vi "LDA_cold_wire_Corr_with_ Displacement.vi"() -> (5 "Plug in titles":string[](array[string]), 7 "Plug in values":string[](array[string]))   [LabVIEW 2016]
uses:
  Globals/Meas_global.vi
  Globals/LDA_meas_global_1.vi
panel:
  in  "Cold Wire":i32=2
  in  "X Displacement (mm)":dbl=4.0
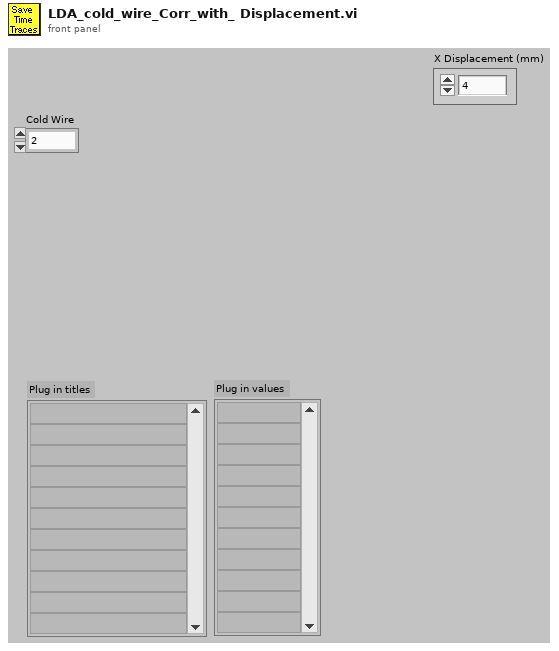
[diagram p1: front panel]
types:
  T1 = typedef "Analysis_info_cluster.ctl" = cluster{"Colour":u32, "Inst type":T2, "Inst name":string, "Symbol":string, "Code name":string, "Extra Info":string, "Inst Array":T3, "Extra Titles":string[], "Extra Values":string[], "U":dbl, "u^2":dbl, "u^3":dbl, "u^4":dbl, "Skew_u":dbl, "Kurt_u":dbl, "Sd Error in Mean":dbl, "% u'/U":dbl, "X":dbl, "Y":dbl, "Z":dbl, "Timescale integral Estimate":dbl, "Sd Error in Variance":dbl, "Calib File":path, "Calib Constants":dbl[], "Output Position":bool, "Full Stats":bool, "Av Sampling Rate":dbl, "Av No of Samples":dbl, "Total Meas Time (s)":dbl, "ADAM Ch Name":string, "Max value":dbl, "Min value":dbl}
  T2 = typedef "Inst_type.ctl" = enum16{"Propeller anemometer", "Raw voltage", "Pressure Transducer", "Pitot-static tube", "Preston tube", "Hot wire", "Cross wire 1", "Cross wire 2", "Generic Linear", "Generic Polynomial", "Generic BackPoly", "Fast FID", "Thermocouple", "Cold wire", "Pulsed Wire", "LDA Vel", "LDA Tran time", "LDA Arr time", "Microphone"}
  T3 = typedef "Instrument_Array.ctl" = enum16{"PWA", "LDA", "Analogue"}
  T4 = typedef "Time_Trace_Cluster.ctl" = cluster{"Weighting":dbl[], "Time (s)":dbl[], "Voltage":dbl[], "Eng Values":dbl[]}
  T5 = typedef "Shift_Cluster.ctl" = cluster{"Stats":dbl[], "Spectra_Auto":dbl[], "Histogram":dbl[], "Hist Max":dbl, "Hist Min":dbl, "No of Samples":i32, "No in plume":i32, "Weight sum":dbl, "No Of Hist bins":i32, "TimeTrace Max":dbl, "Time Trace Min":dbl, "Trace St Deviation":dbl}
  T6 = typedef "Correlation_cluster1.ctl" = cluster{"U inst":string, "uw":dbl, "u^2w":dbl, "uw^2":dbl, "uw/u'w'":dbl, "W inst":string, "uw^3":dbl, "u^3w":dbl, "u^2w^2":dbl, "Index U":i32, "Index W":i32, "Error info":string[]}
  T7 = typedef "Cross_Moments_Shift_Cluster.ctl" = cluster{"Stats":dbl[], "Resampled No of Samples":i32, "Resampled delta T":dbl, "Cross Correlation":dbl[]}
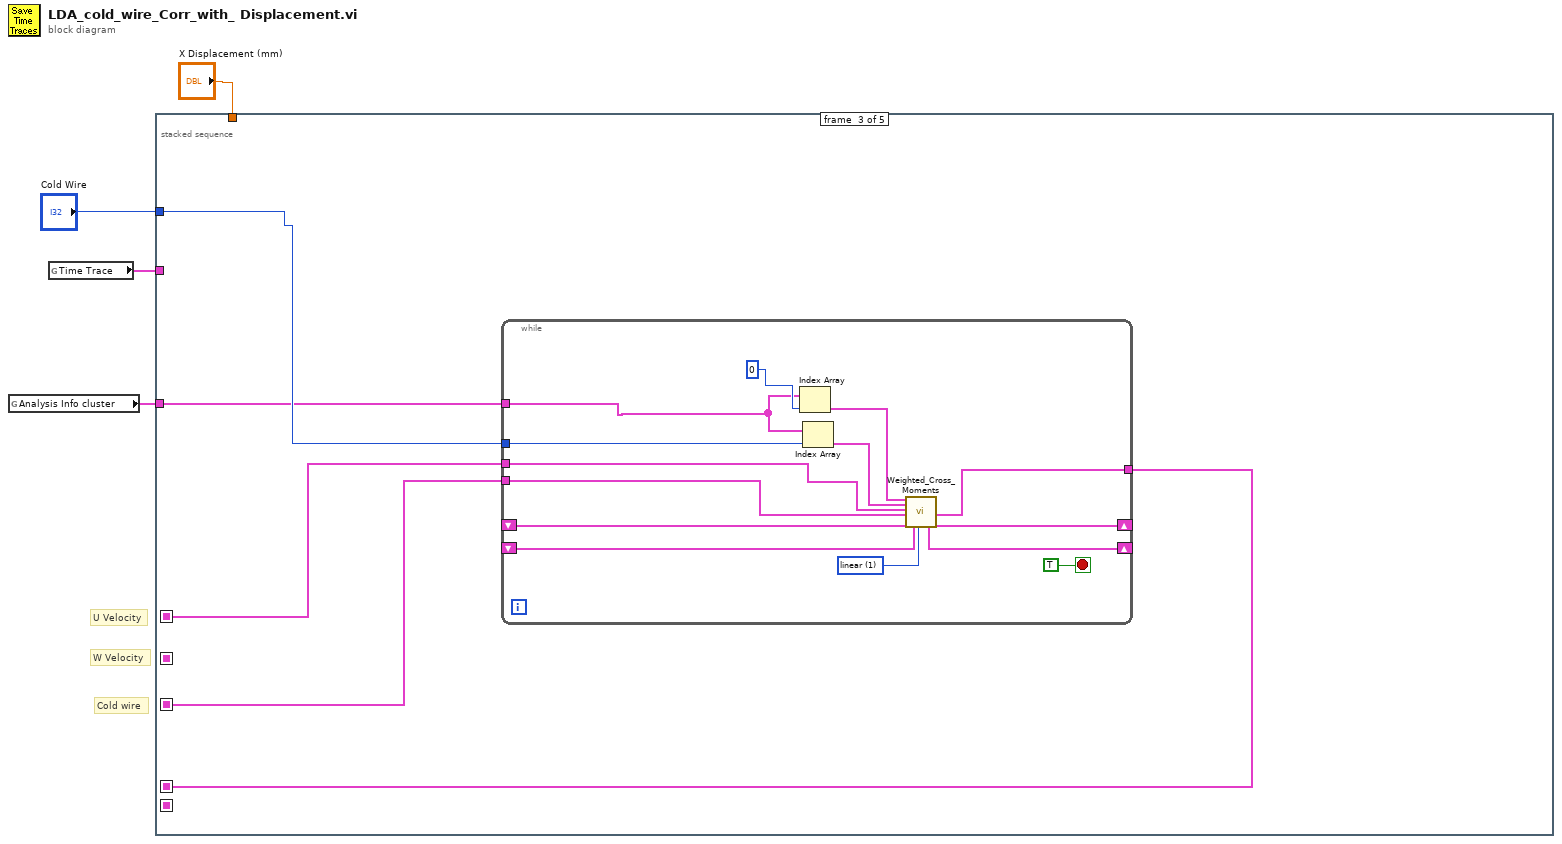
[diagram p0: block diagram]
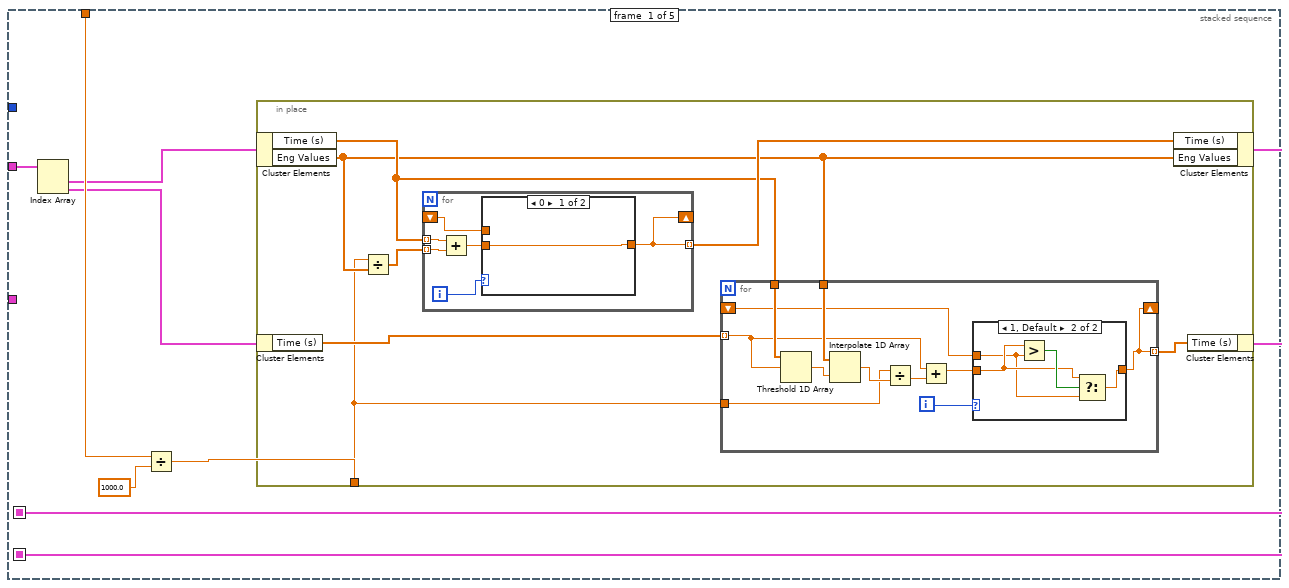
[diagram p2: hidden frame]
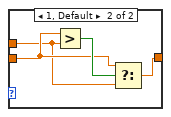
[diagram p3: hidden frame]
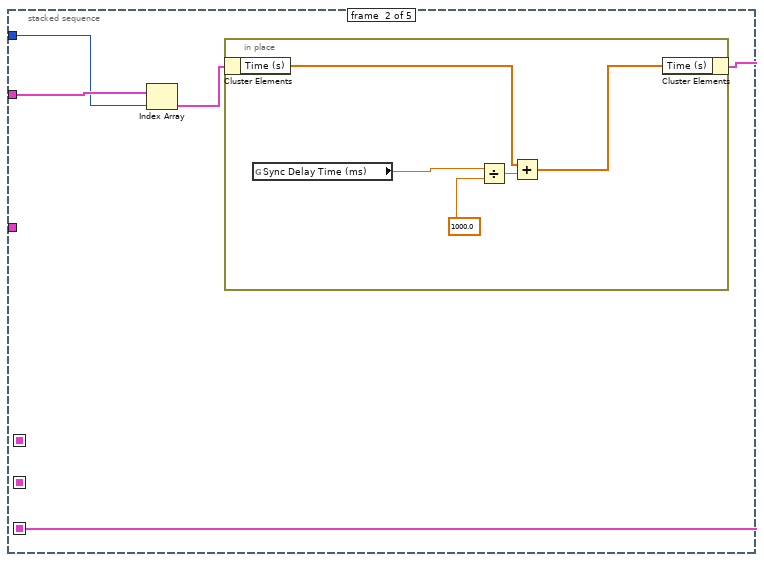
[diagram p5: hidden frame]
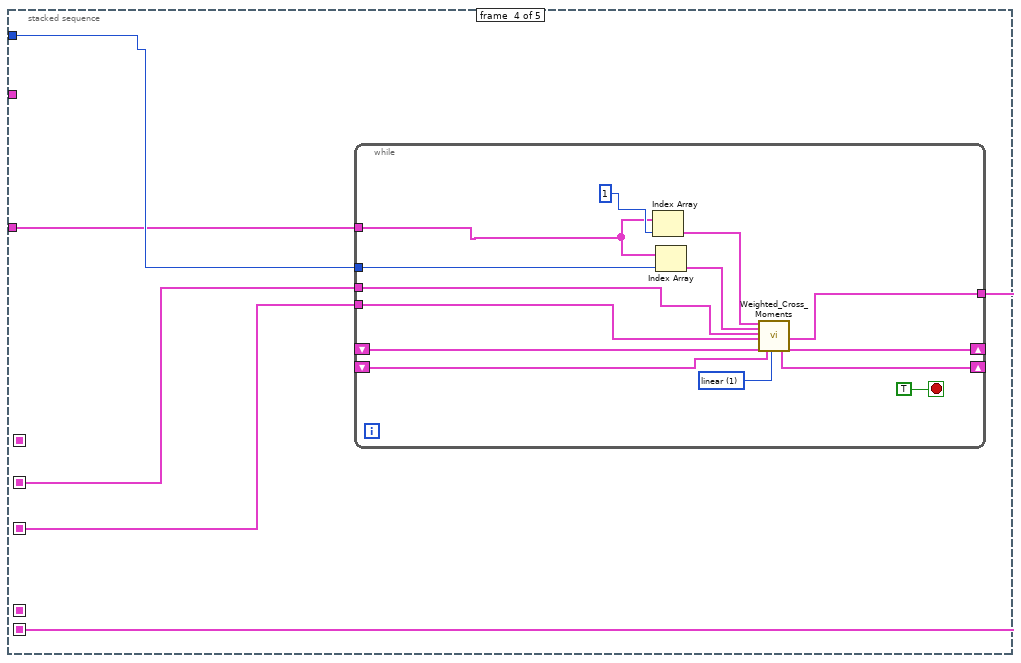
[diagram p6: hidden frame]
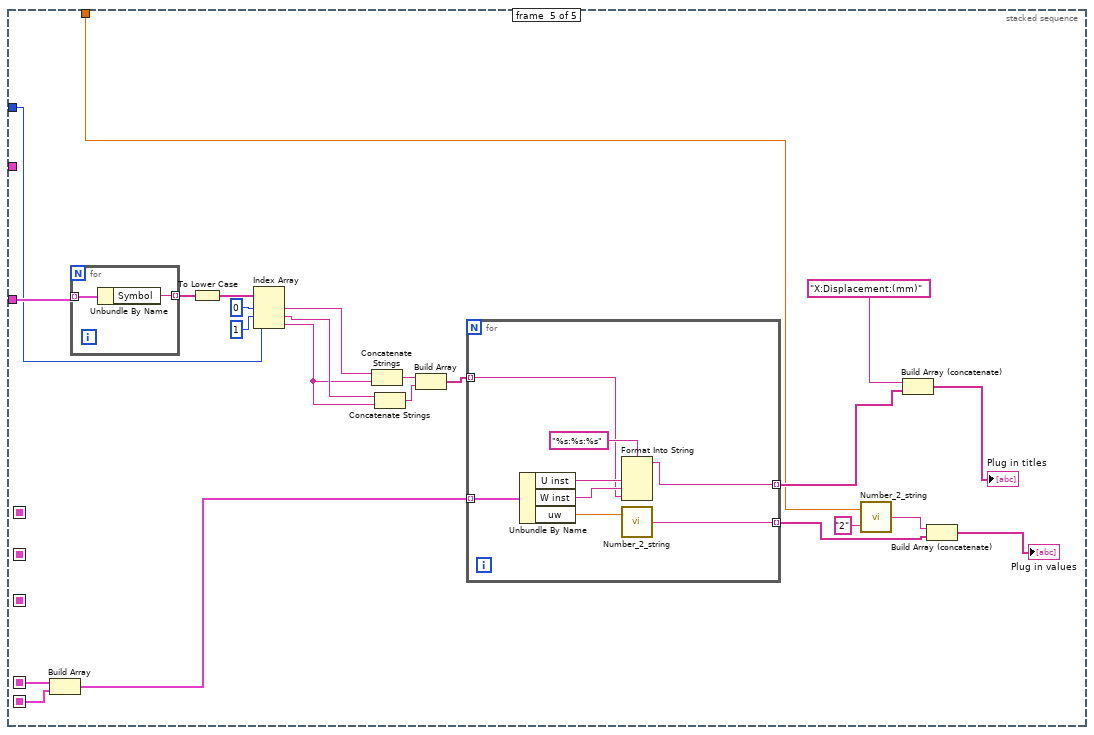
[diagram p7: hidden frame]
diagram:
  # "W Velocity"
  # "Cold wire"
  # "U Velocity"
  n1 = global read "Meas_global.vi" "Analysis Info cluster"() -> (w1:T1[])
  n2 = global read "Meas_global.vi" "Time Trace"() -> (w3:T4[])
  n3 = stacked-sequence {
    seq-local: [w7 _ _ _ _] -> [_ _ w60 _ _]
    seq-local: [_ w48 _ _ _] -> [_ _ w59 w79 _]
    seq-local: [_ _ w57 _ _] -> [_ _ _ _ w115]
    seq-local: [w5 _ _ _ _] -> [_ _ _ w76 _]
    seq-local: [_ _ _ w75 _] -> [_ _ _ _ w116]
    tunnel: "X Displacement (mm)" -> [w12 _ _ _ w95]
    tunnel: w3 -> [w10 w50 _ _ _]
    tunnel: "Cold Wire" -> [_ w47 w58 w78 w110]
    tunnel: w1 -> [_ _ w56 w77 w113]
    frame #0 {
      n4 = Index Array(array=w10) -> (element #1=w9:T4, element #2=w6:T4)  [unwired: 2 in]
      n5 = Divide(x=w12, y=1000.0) -> (x/y=w8:dbl)
      n6 = in-place {
        in-place-border: w8 -> [w15]
        n7 = in-place-cluster #1(w9) -> ("Time (s)"=w18:dbl[], "Eng Values"=w16:dbl[])
        n8 = in-place-cluster #2(w6) -> ("Time (s)"=w17:dbl[])
        n9 = Divide(x=w15, y=w16) -> (x/y=w13:dbl[])
        n10 = for {
          tunnel: w13 -> [w25] mode=indexing
          tunnel: [w21] -> w19 mode=indexing
          tunnel: w18 -> [w24] mode=indexing
          shift-right: [w21] -> _
          shift-left: _ -> [w22]
          i -> [w20]
          n11 = Add(x=w24, y=w25) -> (x+y=w23:dbl)
          n12 = case shown="0" w20 {
            tunnel: w23 -> [w26 w29]
            tunnel: w22 -> [_ w28]
            tunnel: [w26 w27] -> w21
            frame 0 {
            }
            frame 1, Default {
              n13 = Greater?(x=w29, y=w28) -> (0:w30:bool)
              n14 = Select(t=w29, s=w30, f=w28) -> (s? t:f=w27:dbl)
            }
          }
        }
        n15 = for {
          tunnel: w18 -> [w41]
          tunnel: w17 -> [w35] mode=indexing
          tunnel: w16 -> [w40]
          tunnel: w15 -> [w37]
          tunnel: [w32] -> w14 mode=indexing
          shift-right: [w32] -> _
          shift-left: _ -> [w33]
          i -> [w31]
          n16 = Threshold 1D Array(2:w35, 3:w41) -> (0:w39:dbl)  [unwired: 1 in]
          n17 = Interpolate 1D Array(1:w39, 2:w40) -> (0:w38:dbl)
          n18 = Divide(x=w37, y=w38) -> (x/y=w36:dbl)
          n19 = Add(x=w35, y=w36) -> (x+y=w34:dbl)
          n20 = case shown="1, Default" w31 {
            tunnel: w34 -> [w42 w45]
            tunnel: w33 -> [_ w44]
            tunnel: [w42 w43] -> w32
            frame 0 {
            }
            frame 1, Default {
              n21 = Greater?(x=w45, y=w44) -> (0:w46:bool)
              n22 = Select(t=w45, s=w46, f=w44) -> (s? t:f=w43:dbl)
            }
          }
        }
        n23 = in-place-cluster #1("Time (s)"=w19, "Eng Values"=w16) -> (w7:T4)
        n24 = in-place-cluster #2("Time (s)"=w14) -> (w5:T4)
      }
    }
    frame #1 {
      n25 = Index Array(array=w50, index=w47) -> (element=w49:T4)
      n26 = in-place {
        n27 = in-place-cluster #3(w49) -> ("Time (s)"=w51:dbl[])
        n28 = global read "LDA_meas_global_1.vi" "Sync Delay Time (ms)"() -> (w55:dbl)
        n29 = Divide(x=w55, y=1000.0) -> (x/y=w53:dbl)
        n30 = Add(x=w51, y=w53) -> (x+y=w52:dbl[])
        n31 = in-place-cluster #3("Time (s)"=w52) -> (w48:T4)
      }
    }
    frame #2 {
      n32 = while {
        shift-right: [w74] -> _
        shift-left: _ -> [w67]
        tunnel: w60 -> [w69]
        tunnel: w59 -> [w68]
        tunnel: w58 -> [w66]
        tunnel: [w65] -> w57
        tunnel: w56 -> [w64]
        shift-right: [w61] -> _
        shift-left: _ -> [w62]
        stop <- TRUE stop-if-true
        w63 = 1 items=["nearest", "linear", "spline", "cubic Hermite", "Lagrange"] ("interp. method")
        n33 = Index Array(array=w64, index=0) -> (element=w72:T1)
        n34 = Index Array(array=w64, index=w66) -> (element=w71:T1)
        n35 = call "Weighted_Cross_Moments.vi"("AI Cluster 1"=w72, "AI Cluster 2"=w71, "Time Cluster 1"=w69, "Time Cluster 2"=w68, "Shift Cluster In"=w67, "Shift Input"=w62, "interp. method"=w63) -> ("Shift Output"=w61:T5, "output cluster"=w65:T6, "Shift Cluster Out"=w74:T7)  [unwired: 10 in]
      }
    }
    frame #3 {
      n36 = while {
        shift-right: [w93] -> _
        shift-left: _ -> [w86]
        tunnel: w76 -> [w88]
        tunnel: w79 -> [w87]
        tunnel: w78 -> [w85]
        tunnel: [w84] -> w75
        tunnel: w77 -> [w83]
        shift-right: [w80] -> _
        shift-left: _ -> [w81]
        stop <- TRUE stop-if-true
        w82 = 1 items=["nearest", "linear", "spline", "cubic Hermite", "Lagrange"] ("interp. method")
        n37 = Index Array(array=w83, index=1) -> (element=w91:T1)
        n38 = Index Array(array=w83, index=w85) -> (element=w90:T1)
        n39 = call "Weighted_Cross_Moments.vi"("AI Cluster 1"=w91, "AI Cluster 2"=w90, "Time Cluster 1"=w88, "Time Cluster 2"=w87, "Shift Cluster In"=w86, "Shift Input"=w81, "interp. method"=w82) -> ("Shift Output"=w80:T5, "output cluster"=w84:T6, "Shift Cluster Out"=w93:T7)  [unwired: 10 in]
      }
    }
    frame #4 {
      n40 = Build Array(w115, w116) -> (w114:T6[])
      n41 = for {
        tunnel: w113 -> [w118] mode=indexing
        tunnel: [w117] -> w109 mode=indexing
        n42 = Unbundle By Name(w118) -> ("Symbol"=w117:string)
      }
      n43 = To Lower Case(string=w109) -> (all lower case string=w108:string[])
      n44 = Index Array(array=w108, index #1=0 ("index"), index #2=1 ("index"), index #3=w110) -> (element #1=w107:string, element #2=w105:string, element #3=w104:string)
      n45 = Concatenate Strings(w107, w104) -> (w106:string)
      n46 = Concatenate Strings(w105, w104) -> (w103:string)
      n47 = Build Array(w106, w103) -> (w102:string[])
      n48 = for {
        tunnel: [w126] -> w98 mode=indexing
        tunnel: w114 -> [w125] mode=indexing
        tunnel: [w121] -> w100 mode=indexing
        tunnel: w102 -> [w119] mode=indexing
        n49 = Unbundle By Name(w125) -> ("U inst"=w123:string, "W inst"=w122:string, "uw"=w124:dbl)
        n50 = Format Into String(format string="%s:%s:%s", w123, w122, w119) -> (resulting string=w121:string)  [unwired: 2 in, 1 out]
        n51 = call "Number_2_string.vi"("number"=w124) -> ("String"=w126:string)  [unwired: 1 in]
      }
      n52 = call "Number_2_string.vi"("precision"="2", "number"=w95) -> ("String"=w97:string)
      n53 = Build Array (concatenate)("X:Displacement:(mm)", w100) -> (→"Plug in titles":string[])
      n54 = Build Array (concatenate)(w97, w98) -> (→"Plug in values":string[])
    }
  }
